vi "poly_global_eco_plus.vi"(4 "code (w/out ECO)":i32) -> (1 "code (+ ECO)":i32)   [LabVIEW 2015]
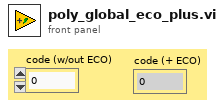
[diagram p1: front panel]
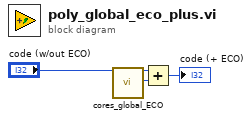
[diagram p0: block diagram]
diagram:
  n1 = call "cores_global_ECO.vi"() -> ("LVutils global ECO"=w1:i32)
  n2 = Add(x="code (w/out ECO)", y=w1) -> (x+y=→"code (+ ECO)":i32)
